vi "peak -- find -- pm - V0.vi"(0 "omega in":dbl[](array[numeric]), 1 "span":dbl=0.01, 2 "z in":cdb[](array[numeric]), 5 "filter method":T5=enum."three", 7 "cursor window":T4={"left"=2378.60310421286, "right "=2421.6740576496672, "center"=2421.6740576496672, "window"=2421.6740576496672, "cursors"=[], "relative"=0, "absolute"=0, "fixed vertical offset"=2421.6740576496672, "vertical offset"=2421.6740576496672, "skew"=2421.6740576496672, "default window frac"=2421.6740576496672, "kind"=enum."fancy", "skew.left"=2421.6740576496672, "skew.right"=0.0, "Plot ref"=refnum, "wing order"=enum."back"}, 12 "plots: filter related":T1) -> (4 "center":cdb=0.005233304275841307+0.002092688467219436i, 15 "lorentzian":T2={"Amplitude"=-1.0311345636926572, "omega(0)"=-1.0311345636926572, "Gamma"=-1.0311345636926572, "phase"=-1.0311345636926572, "Q"=-1.0311345636926572, "Norm  Ampl"=-1.0311345636926572, "z (inf)"=-1.0311345636926572+0.0i, "4corners"={"z (-pi/2)"=-1.0311345636926572+0.5736824521422934i, "z(inf)"=-0.5200164984937075+1.0975277942502903i, "z (pi/2)"=-1.0311345636926572+0.5736824521422934i, "z center"=-0.5136528600391839+0.580046090596817i, "z(0)"=-0.5200164984937075+1.0975277942502903i, "radius"=-1.0311345636926572}} {"z (inf)" format="%#9_9f"; "Q" format="%#9_9f"; "phase" format="%#9_9f"; "Gamma" format="%#9_9f"; "omega(0)" format="%#9_9f"})   [LabVIEW 2010]
uses:
  filter method control.ctl
  cursor winow.ctl
  lorentzian.ctl
  circle corners.ctl
  plot refs -- filter related.ctl
  tale of three indices.vi
  containing bix.vi
  Q -- check range -- i -- real.vi
  filter -- window span logic.vi
  linear interp iiii- complex - z-omega - divide.vi
  linear interpolation iiii- complex.vi
  command stack.vi
  tale of three indices -- check state.vi
  Q -- check range -- i -- integer.vi
  Q - not nan -- real.vi
  linear interp iiii- complex - z-omega.vi
  line -- complex.vi
  Q - not nan -- integer.vi
  <vilib>/Analysis/Matrix/Numeric/Conversions/Array To Matrix.vi
  <vilib>/Analysis/Matrix/Numeric/Conversions/Array To Matrix - RA2.vi
  <vilib>/Analysis/baseanly.llb/Inverse Matrix.vi
  <vilib>/Analysis/baseanly.llb/Real Inverse Matrix.vi
  <vilib>/analysis/baseanly.llb/A x B.vi
  <vilib>/Analysis/baseanly.llb/Complex A x B.vi
panel:
  in  "Plot: phase":refnum<vi>
  in  "Plot: win omega":refnum<vi>
  in  "Plot: fragment":refnum<vi>
  in  "Plot: dz/domega":refnum<vi>
  in  "Plot: complex plane - filter":refnum<vi>
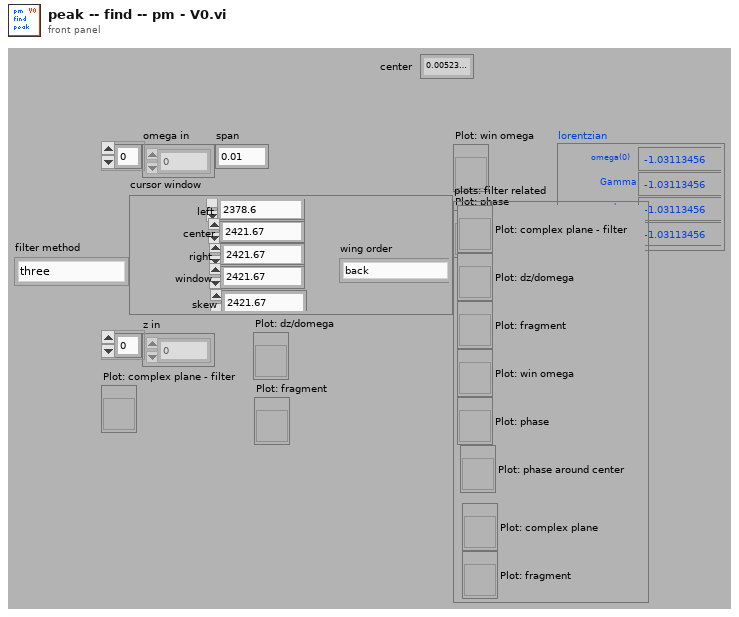
[diagram p1: front panel]
types:
  T1 = typedef "plot refs -- filter related.ctl" = cluster{"Plot: complex plane - filter":refnum<vi>, "Plot: dz/domega":refnum<vi>, "Plot: fragment":refnum<vi>, "Plot: win omega":refnum<vi>, "Plot: phase":refnum<vi>, "Plot: phase around center":refnum<vi>, "Plot: complex plane":refnum<vi>, "Plot: fragment":refnum<vi>}
  T2 = typedef "lorentzian.ctl" = cluster{"Amplitude":dbl, "omega(0)":dbl, "Gamma":dbl, "phase":dbl, "Q":dbl, "Norm  Ampl":dbl, "z (inf)":cdb, "4corners":T3}
  T3 = typedef "circle corners.ctl" = cluster{"z (-pi/2)":cdb, "z(inf)":cdb, "z (pi/2)":cdb, "z center":cdb, "z(0)":cdb, "radius":dbl}
  T4 = typedef "cursor winow.ctl" = cluster{"left":dbl, "right ":dbl, "center":dbl, "window":dbl, "cursors":i32[], "relative":i32, "absolute":i32, "fixed vertical offset":dbl, "vertical offset":dbl, "skew":dbl, "default window frac":dbl, "kind":enum16{"symmetric", "skewed", "fancy"}, "skew.left":dbl, "skew.right":dbl, "Plot ref":refnum<vi>, "wing order":enum16{"forw", "back"}}
  T5 = typedef "filter method control.ctl" = enum16{"four", "five", "one", "two", "three", "zero", "minus one", "minus two"}
  T6 = typedef "tale of three indices -- int -- control.ctl" = cluster{"left":i32, "center":i32, "right":i32, "right most":i32, "left most":i32, "window":i32, "max win factor":i32, "max win":i32, "min win":i32}
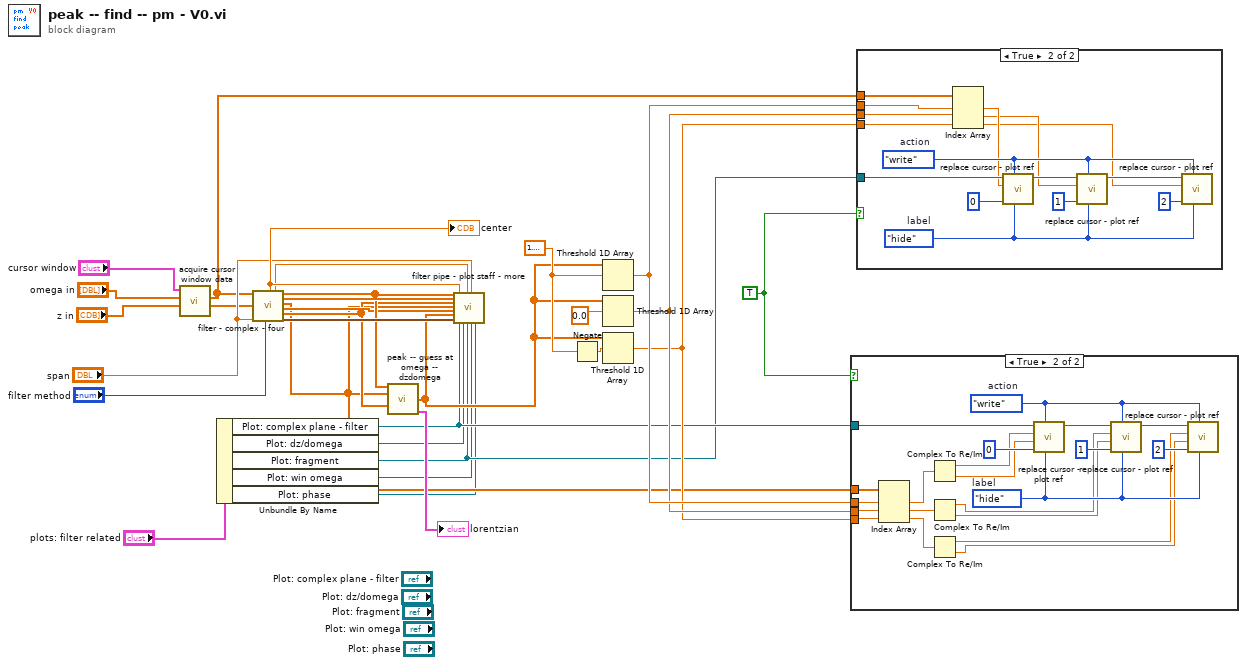
[diagram p0: block diagram]
diagram:
  w9 = TRUE
  w16 = 1.5707963267948966
  n1 = call "acquire cursor window data.vi"("z in"="z in", "omega in"="omega in", "cursor window"="cursor window") -> ("z out"=w14:cdb[], "omega  out"=w15:dbl[])  [unwired: 4 in, 3 out]
  n2 = Unbundle By Name("plots: filter related") -> ("Plot: complex plane - filter"=w6:refnum<vi>, "Plot: dz/domega"=w5:refnum<vi>, "Plot: fragment"=w4:refnum<vi>, "Plot: win omega"=w3:refnum<vi>, "Plot: phase"=w2:refnum<vi>)
  n3 = call "filter - complex - four.vi"("omega  in"=w15, "z in"=w14, "span"="span", "filter method"="filter method") -> ("center"=w23:cdb, "norm"=w22:dbl, "omega out"=w24:dbl[], "z in out"=w27:cdb[], "z out"=w8:cdb[], "win omega out"=w20:dbl[], "dz/domega out"=w19:cdb[], "tale of three"=w28:T6)  [unwired: 8 in]
  "center" <- w23
  n4 = call "peak -- guess at omega -- dzdomega.vi"("omega"=w24, "z"=w8, "dz/domega"=w19) -> ("theta"=w7:dbl[], "pm lorentzian"=→"lorentzian":T2)  [unwired: 8 in, 3 out]
  n5 = call "filter pipe - plot staff - more.vi"("omega  in"=w24, "zin"=w27, "dz/domega in"=w19, "z out"=w8, "win omega"=w20, "phase"=w7, "tale of three indices -- int -- control"=w28, "center"=w23, "Plot: complex plane - filter"=w6, "Plot: dz/domega"=w5, "norm"=w22, "Plot: fragment"=w4, "smart filter: span"="span", "Plot: win omega"=w3, "Plot: phase"=w2) -> ()  [unwired: 13 in]
  n6 = Negate(x=w16) -> (-x=w10:dbl)
  n7 = Threshold 1D Array(2:w16, 3:w7) -> (0:w13:dbl)  [unwired: 1 in]
  n8 = Threshold 1D Array(2:0.0 ("threshold y"), 3:w7) -> (0:w12:dbl)  [unwired: 1 in]
  n9 = Threshold 1D Array(2:w10, 3:w7) -> (0:w11:dbl)  [unwired: 1 in]
  n10 = case shown="True" w9 {
    tunnel: w6 -> [_ w44]
    tunnel: w8 -> [_ w34]
    tunnel: w13 -> [_ w33]
    tunnel: w12 -> [_ w32]
    tunnel: w11 -> [_ w31]
    frame False {
    }
    frame True {
      w45 = enum16{"hide", "show x", "show y", "show (x,y)"}."hide"  # label
      w51 = enum16{"", "read", "write"}."write"  # action
      n11 = Index Array(array=w34, index #1=w33, index #2=w32, index #3=w31) -> (element #1=w41:cdb, element #2=w42:cdb, element #3=w43:cdb)
      n12 = Complex To Re/Im(x + iy=w41) -> (x=w40:dbl, y=w39:dbl)
      n13 = Complex To Re/Im(x + iy=w42) -> (x=w38:dbl, y=w37:dbl)
      n14 = Complex To Re/Im(x + iy=w43) -> (x=w36:dbl, y=w35:dbl)
      n15 = call "replace cursor - plot ref.vi"("label"=w45, "action"=w51, "cursor index"=0, "new  Y"=w39, "new X"=w40, "Plot ref in"=w44) -> ("Plot ref out"=w47:refnum<vi>)  [unwired: 3 in, 2 out]
      n16 = call "replace cursor - plot ref.vi"("label"=w45, "action"=w51, "cursor index"=1, "new  Y"=w37, "new X"=w38, "Plot ref in"=w47) -> ("Plot ref out"=w46:refnum<vi>)  [unwired: 3 in, 2 out]
      n17 = call "replace cursor - plot ref.vi"("label"=w45, "action"=w51, "cursor index"=2, "new  Y"=w35, "new X"=w36, "Plot ref in"=w46) -> ()  [unwired: 3 in, 3 out]
    }
  }
  n18 = case shown="True" w9 {
    tunnel: w4 -> [_ w59]
    tunnel: w13 -> [_ w55]
    tunnel: w12 -> [_ w54]
    tunnel: w11 -> [_ w53]
    tunnel: w15 -> [_ w52]
    frame False {
    }
    frame True {
      w60 = enum16{"hide", "show x", "show y", "show (x,y)"}."hide"  # label
      w66 = enum16{"", "read", "write"}."write"  # action
      n19 = Index Array(array=w52, index #1=w55, index #2=w54, index #3=w53) -> (element #1=w58:dbl, element #2=w57:dbl, element #3=w56:dbl)
      n20 = call "replace cursor - plot ref.vi"("label"=w60, "action"=w66, "cursor index"=0, "new X"=w58, "Plot ref in"=w59) -> ("Plot ref out"=w62:refnum<vi>)  [unwired: 4 in, 2 out]
      n21 = call "replace cursor - plot ref.vi"("label"=w60, "action"=w66, "cursor index"=1, "new X"=w57, "Plot ref in"=w62) -> ("Plot ref out"=w61:refnum<vi>)  [unwired: 4 in, 2 out]
      n22 = call "replace cursor - plot ref.vi"("label"=w60, "action"=w66, "cursor index"=2, "new X"=w56, "Plot ref in"=w61) -> ()  [unwired: 4 in, 3 out]
    }
  }
